vi "Offset status-deduce condition.vi"(8 "error in (no error)":errorcluster, 9 "Z_offset":bool, 10 "Y_offset":bool, 11 "X_offset":bool) -> (0 "error out":errorcluster, 3 "Status":T1(ring))   [LabVIEW 2020]
panel:
  out "Number 2":u32 format="%b"
  out "Array":bool[](array[boolean])
  out "Number":u32
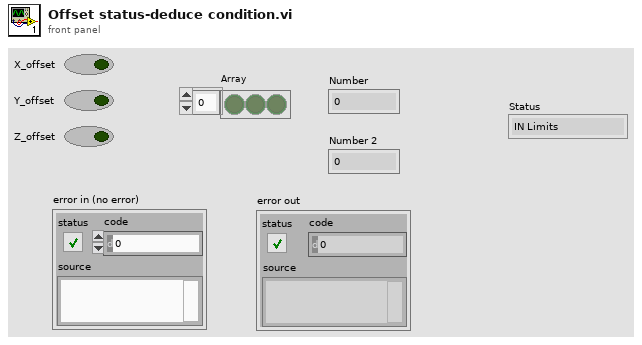
[diagram p1: front panel]
types:
  T1 = enum16{"IN Limits", "X/Y Exceeded", "Z Exceeded", "X/Y & Z Exceeded"}
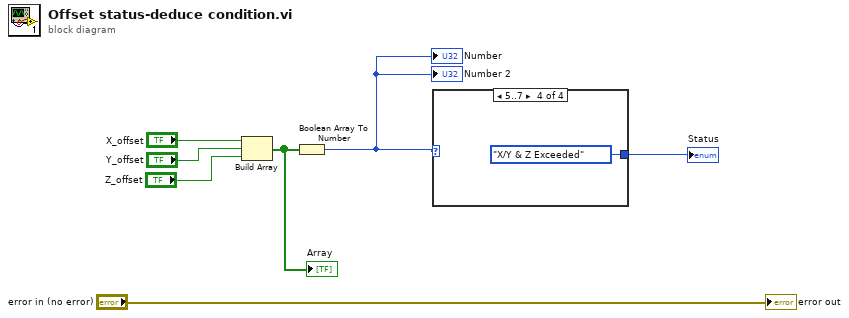
[diagram p0: block diagram]
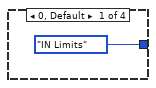
[diagram p2: hidden frame]
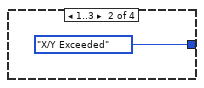
[diagram p3: hidden frame]
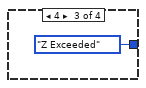
[diagram p4: hidden frame]
diagram:
  n1 = Build Array("X_offset", "Y_offset", "Z_offset") -> (w3:bool[])
  "Array" <- w3
  n2 = Boolean Array To Number(Boolean array=w3) -> (number=w2:u32)
  "Number" <- w2
  "Number 2" <- w2
  n3 = case shown="5..7" w2 {
    tunnel: [T1."IN Limits" ("Status") T1."X/Y Exceeded" ("Status") T1."Z Exceeded" ("Status") T1."X/Y & Z Exceeded" ("Status")] -> w1
    frame 0, Default {
    }
    frame 1..3 {
    }
    frame 4 {
    }
    frame 5..7 {
    }
  }
  "Status" <- w1
  "error out" <- "error in (no error)"
